vi "ConfigurationInputOutput.vi"(0 "EpiWrapper in":refnum<class "EpiWrapper.lvclass">, 1 "Action":enum16{"Read", "Write"}(ring), 2 "error in (no error)":errorcluster) -> (3 "EpiWrapper out":refnum<class "EpiWrapper.lvclass">, 4 "error?":bool, 5 "message":string, 6 "error out":errorcluster)   [LabVIEW 2012, in "EpiWrapper.lvclass"]
uses:
  EpiWrapper.lvclass
  <vilib>/Utility/error.llb/DialogType.ctl
  EpiWrapper.lvclass/EpiWrapper.ctl
  <vilib>/Utility/config.llb/Read Key (I32).vi
  <vilib>/Utility/config.llb/Read Key (Double).vi
  <vilib>/Utility/config.llb/Write Key (I32).vi
  <vilib>/Utility/config.llb/Write Key (Double).vi
  <vilib>/Utility/config.llb/NI_LVConfig.lvlib
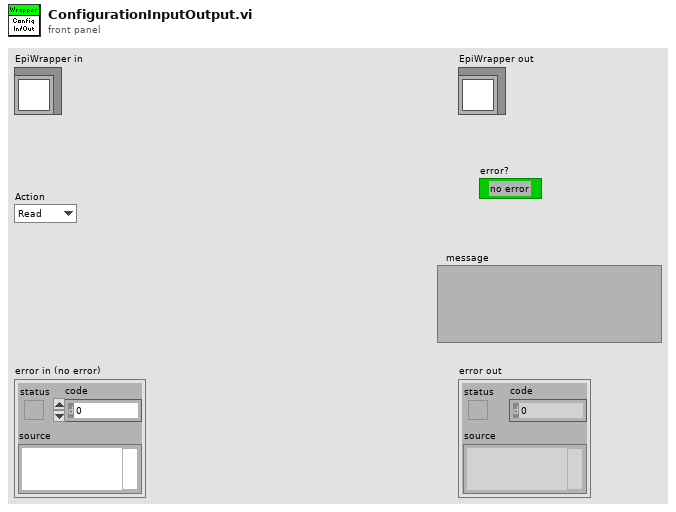
[diagram p1: front panel]
types:
  T1 = typedef "DialogType.ctl" = u16
  T2 = typedef "AppPaths.ctl" = cluster{"DataDir":T3, "OmniDriver":T3, "OmniDriverCommon":T3, "Configuration":T3, "WaferImage":T3}
  T3 = typedef "PathTraveler.ctl" = cluster{"Enum":T4, "FileName":string, "Exists?":bool, "Path":path}
  T4 = typedef "PathTypes.ctl" = enum16{"DataDir", "OmniDriver", "OmniDriver_Common", "Configuration", "WaferImage"}
  T5 = typedef "NI_LVConfig.lvlib/Config Data RefNum.ctl" = refnum<k1>
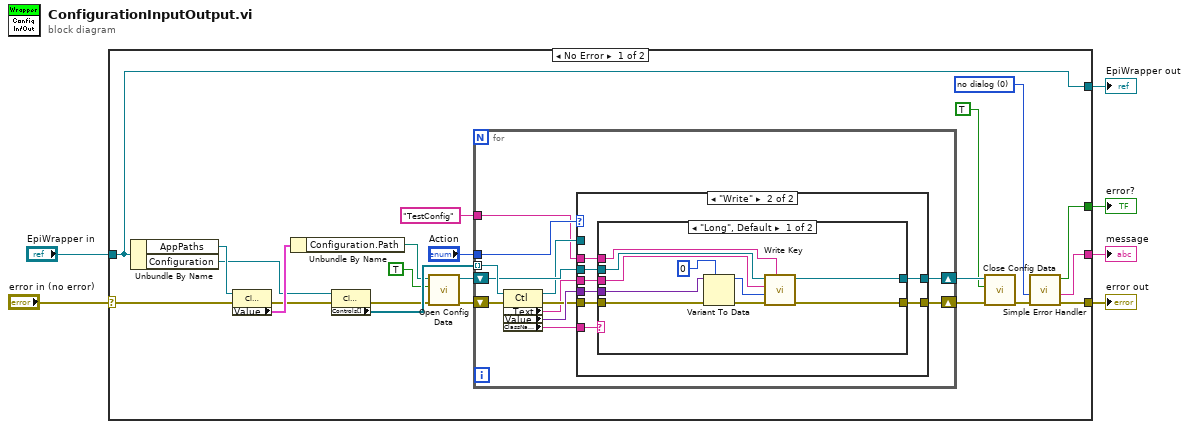
[diagram p0: block diagram]
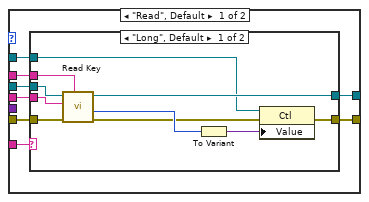
[diagram p2: hidden frame]
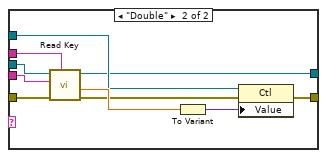
[diagram p3: hidden frame]
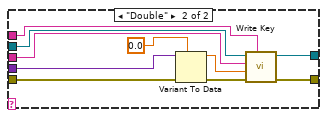
[diagram p4: hidden frame]
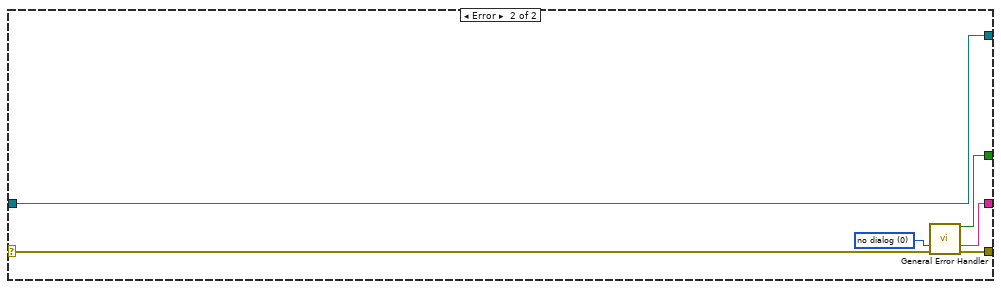
[diagram p5: hidden frame]
diagram:
  n1 = case shown="No Error" "error in (no error)" {
    selector: "error in (no error)" -> [w13 w101]
    tunnel: [w10 w99] -> w5
    tunnel: [w9 w102] -> w3
    tunnel: "EpiWrapper in" -> [w9 w102]
    tunnel: [w12 w97] -> w2
    tunnel: [w11 w98] -> w1
    frame No Error {
      w20 = T1 0 items=["no dialog", "OK message", "continue or stop message", "OK message + warnings", "continue/stop + warnings"] ("type of dialog (OK msg:1)")
      n2 = Unbundle By Name(w9) -> ("AppPaths"=w18:refnum<vi>, "Configuration"=w15:refnum<vi>)
      n3 = property class="Clust (strict)"(reference=w18, error in=w13) -> (error out=w14:errorcluster, "Value"=w17:T2)  [unwired: 1 out]
      n4 = Unbundle By Name(w17) -> ("Configuration.Path"=w16:path)
      n5 = property class="Clust (strict)"(reference=w15, error in=w14) -> (error out=w7:errorcluster, "Controls[]"=w19:refnum<vi>[])  [unwired: 1 out]
      n6 = call <vilib>:"Open Config Data.vi"("error in (no error)"=w7, "create file if necessary (T)"=TRUE, "configuration file path"=w16) -> ("error out"=w27:errorcluster, "refnum"=w28:T5)  [unwired: 6 in, 1 out]
      n7 = for {
        tunnel: w19 -> [w40] mode=indexing
        shift-right: [w35] -> w24
        shift-left: w27 -> [w36]
        shift-right: [w34] -> w26
        shift-left: w28 -> [w37]
        tunnel: "Action" -> [w33]
        tunnel: "TestConfig" ("section") -> [w31]
        n8 = property class="Ctl"(reference=w40, error in=w36) -> (reference out=w32:refnum<vi>, error out=w38:errorcluster, "Label.Text"=w29:string, "Value"=w39:variant, "ClassName"=w30:string)
        n9 = case shown="\"Write\"" w33 {
          tunnel: w39 -> [_ w76]
          tunnel: w38 -> [w47 w75]
          tunnel: w37 -> [w48 w74]
          tunnel: [w45 w73] -> w35
          tunnel: [w44 w72] -> w34
          tunnel: w32 -> [w46 _]
          tunnel: w31 -> [w42 w71]
          tunnel: w30 -> [w43 w70]
          tunnel: w29 -> [w41 w69]
          frame "Read", Default {
            n10 = case shown="\"Long\", Default" w43 {
              tunnel: [w51 w61] -> w45
              tunnel: [w56 w62] -> w44
              tunnel: w48 -> [w58 w65]
              tunnel: w47 -> [w57 w63]
              tunnel: w46 -> [w53 w64]
              tunnel: w42 -> [w50 w60]
              tunnel: w41 -> [w49 w59]
              frame "Long", Default {
                n11 = call-poly <vilib>:"Read Key.vi"("section"=w50, "error in (no error)"=w57, "key"=w49, "refnum"=w58) -> ("error out"=w52:errorcluster, "value"=w54:i32, "refnum out"=w56:T5)  [unwired: 1 in, 4 out]
                n12 = To Variant(anything=w54) -> (Variant=w55:variant)
                n13 = property class="Ctl"(reference=w53, error in=w52, "Value"=w55) -> (error out=w51:errorcluster)  [unwired: 1 out]
              }
              frame "Double" {
                n14 = call-poly <vilib>:"Read Key.vi"("section"=w60, "error in (no error)"=w63, "key"=w59, "refnum"=w65) -> ("error out"=w66:errorcluster, "value"=w67:dbl, "refnum out"=w62:T5)  [unwired: 1 in, 4 out]
                n15 = To Variant(anything=w67) -> (Variant=w68:variant)
                n16 = property class="Ctl"(reference=w64, error in=w66, "Value"=w68) -> (error out=w61:errorcluster)  [unwired: 1 out]
              }
            }
          }
          frame "Write" {
            n17 = case shown="\"Long\", Default" w70 {
              tunnel: w76 -> [w86 w95]
              tunnel: w75 -> [w84 w94]
              tunnel: [w81 w90] -> w73
              tunnel: w74 -> [w80 w91]
              tunnel: [w79 w89] -> w72
              tunnel: w71 -> [w78 w88]
              tunnel: w69 -> [w77 w87]
              frame "Long", Default {
                n18 = Variant To Data(error in=w84, type=0, Variant=w86) -> (data=w83:i32, error out=w82:errorcluster)
                n19 = call-poly <vilib>:"Write Key.vi"("section"=w78, "error in (no error)"=w82, "value"=w83, "key"=w77, "refnum"=w80) -> ("error out"=w81:errorcluster, "refnum out"=w79:T5)  [unwired: 4 in, 1 out]
              }
              frame "Double" {
                n20 = Variant To Data(error in=w94, type=0.0, Variant=w95) -> (data=w93:dbl, error out=w92:errorcluster)
                n21 = call-poly <vilib>:"Write Key.vi"("section"=w88, "error in (no error)"=w92, "value"=w93, "key"=w87, "refnum"=w91) -> ("error out"=w90:errorcluster, "refnum out"=w89:T5)  [unwired: 4 in, 1 out]
              }
            }
          }
        }
      }
      n22 = call <vilib>:"Close Config Data.vi"("error in (no error)"=w24, "write file if changed (T)"=TRUE, "refnum"=w26) -> ("error out"=w21:errorcluster)  [unwired: 8 out]
      n23 = call <vilib>:"Simple Error Handler.vi"("type of dialog (OK msg:1)"=w20, "error in (no error)"=w21) -> ("error?"=w12:bool, "source out"=w11:string, "error out"=w10:errorcluster)  [unwired: 3 in, 2 out]
    }
    frame Error {
      w100 = T1 0 items=["no dialog", "OK message", "continue or stop message", "OK message + warnings", "continue/stop + warnings"] ("type of dialog (OK msg:1)")
      n24 = call <vilib>:"General Error Handler.vi"("type of dialog (OK msg:1)"=w100, "error in (no error)"=w101) -> ("error?"=w97:bool, "message"=w98:string, "error out"=w99:errorcluster)  [unwired: 9 in, 2 out]
    }
  }
  "error out" <- w5
  "EpiWrapper out" <- w3
  "error?" <- w2
  "message" <- w1
